vi "Check AI IRQ.vi"(5 "Hysteresis":u16, 6 "FIFO In":refnum<k21>="IRQ Queue", 7 "IRQ Number":u8, 8 "Threshold":u16, 9 "Analog Value":u16, 10 "Rising Edge?":bool, 11 "Enable Interrupt?":bool) -> ()   [LabVIEW 2017]
doc: "This VI checks if the analog input interrupt is triggered under the specified condition.\n<b>IRQ Number</b> specifies the identifier of the interrupt. <b>IRQ Number</b> ranges from 1 to 8 on FPGA and is shared between analog, digital, and button interrupts."
uses:
  <vilib>/Platform/TimedLoop/XDataNode/timing_clust.ctl
  <vilib>/Platform/TimedLoop/XDataNode/nitl_modes.ctl
  <vilib>/Platform/TimedLoop/XDataNode/wakeup.ctl
  <vilib>/rvi/Emulation/niFpgaSctlEmulationGetInTimedLoop.vi
  <vilib>/rvi/Emulation/niFpgaEmulationReportErrorSimple.vi
  <vilib>/rvi/Emulation/niFpgaGetClockAttributes.vi
  <vilib>/rvi/Emulation/niFpgaCriticalErrorInLSC.vi
  <vilib>/rvi/DataTransferAndStorage/Container/Common/niFpgaContainerExecOnDevCompGetState.vi
  <vilib>/rvi/Emulation/niFpgaEmulationIsFPGAContextNoSignature.vi
  <vilib>/rvi/errors/niFpgaSetErrorForExecOnDevCompSimple.vi
  <vilib>/rvi/eio/common/nirviEmuReportErrorAndStop.vi
  <vilib>/rvi/DataTransferAndStorage/Container/Common/niFpgaContainerGetUniqueNameForEmu.vi
  <vilib>/rvi/FIFO/Fifo_Resource/nirvififoEmulationSetSize.vi
  <vilib>/rvi/FIFO/Fifo_Resource/nirviFifoEmulationQueueMgr.vi
  <instcachedir>/0/nirviFifoEmulationQueueMgr_E5CAEC123FF24DC58D834DCA3CDAA9B5.lvgen/nirviFifoEmulationQueueMgr_E5CAEC123FF24DC58D834DCA3CDAA9B5_001.vi
  <vilib>/rvi/FIFO/Fifo_Resource/nirvififoEmulationDetermineInputValidOut.vi
  <vilib>/rvi/FIFO/Fifo_Resource/nirvififoEmulationCreateLock.vi
  <vilib>/rvi/Emulation/niFpgaProcessEmulError.vi
  <vilib>/rvi/FIFO/Fifo_Resource/nirvififoEmulationObtainLock.vi
  <vilib>/rvi/FIFO/Fifo_Resource/nirvififoEmulationReleaseLock.vi
  <vilib>/rvi/occurrence/nirviWaitOnOccurrenceBase.vi
  <vilib>/rvi/errors/nirviReportUnexpectedCaseInternalError.vi
  <vilib>/rvi/errors/nirviReportUnexpectedCaseInternalError (U32).vi
  <vilib>/Utility/error.llb/Clear Errors.vi
  <vilib>/rvi/interface/RandomDataEmulation/niFpgaRandomDataHandleErrors.vi
  <vilib>/platform/TimedLoop/XDataNode/XDataNode.xnode
  <vilib>/rvi/DataTransferAndStorage/Container/XNode/niFpgaContainer.xnode
  <vilib>/rvi/FIFO/Fifo_Resource/niFpgaFifoEmulationRefIn.vi
  <vilib>/Platform/TimedLoop/XDataNode/XDNodeRunTimeDep.lvlib
panel:
  # "This VI checks if the analog input interrupt is triggered under the specified condition.\nIRQ Number specifies the identifier of the interrupt. IRQ Number ranges from 1 to 8 on FPGA and is shared between analog, digital, and button interrupts."
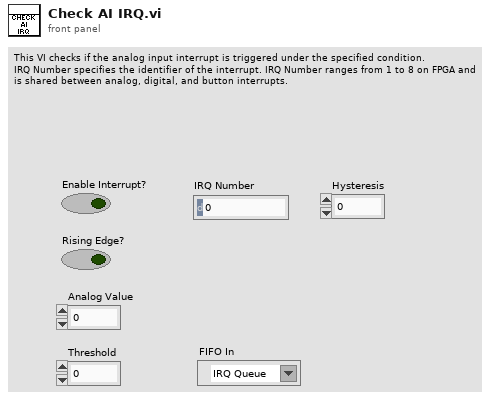
[diagram p1: front panel]
types:
  T1 = typedef "XDNodeRunTimeDep.lvlib/timing_clust.ctl" = cluster{"Expected End [f-1]":u64, "Actual End [f-1]":u64, "Finished Late? [f-1]":bool, "Expected End [i-1]":u64, "Actual End [i-1]":u64, "Finished Late? [i-1]":bool, "Expected Start [i]":u64, "Actual Start [i]":u64, "Expected Start [f]":u64, "Actual Start [f]":u64, "Source Name":string, "Structure Name":string, "Period":i64, "Deadline":i64, "Offset":i64, "Start":i64, "Priority":i32, "Timeout":i32, "Mode":T2, "Wakeup Reason":T3, "Error":errorcluster, "Source Type":string, "Secondary Source Type":string, "Global End Time":u64, "Global Start Time":u64, "Frame Duration":u64, "Iteration Duration":u64, "Assigned CPU":i32, "I/O Scan Engine Mode":u32}
  T2 = typedef "XDNodeRunTimeDep.lvlib/nitl_modes.ctl" = enum32{"No Change", "Process missed periods, maintain original phase", "Discard missed periods, maintain original phase", "Process missed periods, ignore original phase", "Discard missed periods, ignore original phase"}
  T3 = typedef "XDNodeRunTimeDep.lvlib/wakeup.ctl" = enum32{"Normal", "Aborted", "Asynchronous wakeup", "Timing source error", "Timed loop error", "Timeout"}
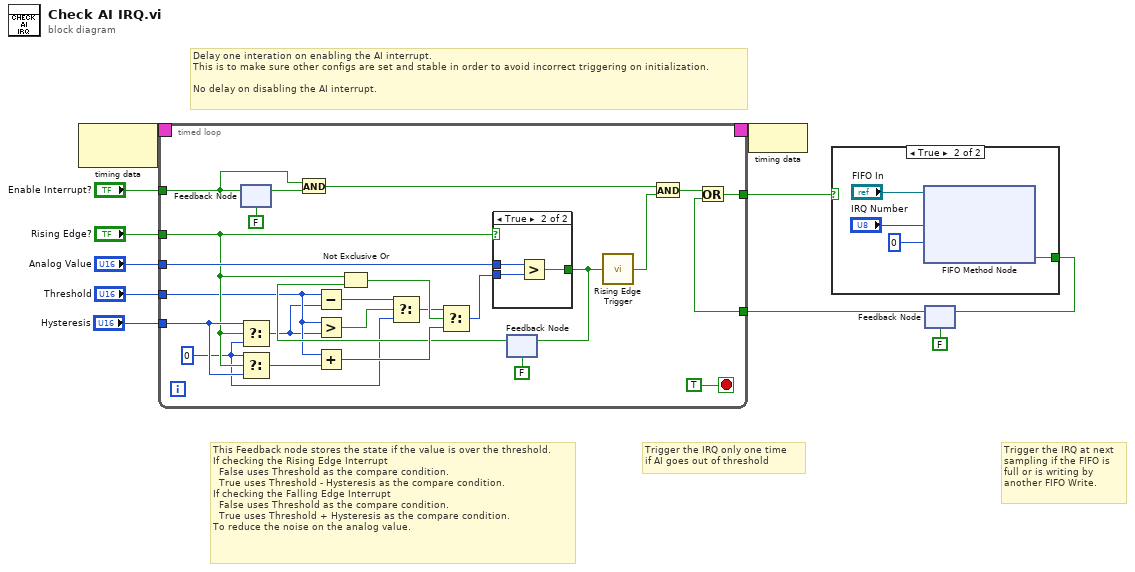
[diagram p0: block diagram]
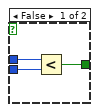
[diagram p2: hidden frame]
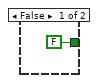
[diagram p3: hidden frame]
diagram:
  # "Delay one interation on enabling the AI interrupt.\nThis is to make sure other configs are set and stable in order to avoid incorrect triggering on initialization.\n\nNo delay on disabling the AI interrupt."
  # "Trigger the IRQ only one time \nif AI goes out of threshold"
  # "This Feedback node stores the state if the value is over the threshold.\nIf checking the Rising Edge Interrupt\n  False uses Threshold as the compare condition.\n  True uses Threshold - Hysteresis as the compare condition.\nIf checking the Falling Edge Interrupt\n  False uses Threshold as the compare condition.\n  True uses Threshold + Hysteresis as the compare condition.\nTo reduce the noise on the analog value."
  # "Trigger the IRQ at next \nsampling if the FIFO is \nfull or is writing by \nanother FIFO Write."
  n1 = node-c288() -> (w7:T1)  [unwired: 1 in]
  n2 = feedback #1(FALSE ("Timed Out?")) -> (w2:bool)
  n3 = timed-loop {
    timing: w7 -> [_]
    timing-out: [_] -> w6
    tunnel: "Analog Value" -> [w36]
    tunnel: "Threshold" -> [w23]
    tunnel: "Hysteresis" -> [w26]
    tunnel: "Rising Edge?" -> [w25]
    tunnel: [w28] -> w3
    tunnel: w2 -> [w27]
    tunnel: "Enable Interrupt?" -> [w15]
    stop <- TRUE stop-if-true
    w18 = u16 0 ("f")
    n4 = feedback-in #2(w15) -> ()
    n5 = feedback #2(FALSE ("Enable Interrupt?")) -> (w14:bool)
    n6 = Select(t=w26, s=w25, f=w18) -> (s? t:f=w22:u16)
    n7 = Select(t=w18, s=w25, f=w26) -> (s? t:f=w24:u16)
    n8 = And(x=w15, y=w14) -> (x .and. y?=w13:bool)
    n9 = Subtract(x=w23, y=w22) -> (x-y=w20:u16)
    n10 = Greater?(x=w23, y=w22) -> (0:w21:bool)
    n11 = Add(x=w23, y=w24) -> (x+y=w34:u16)
    n12 = Select(t=w20, s=w21, f=w18) -> (s? t:f=w19:u16)
    n13 = feedback #3(FALSE ("Timed Out?")) -> (w31:bool)
    n14 = Not Exclusive Or(1:w31, 2:w25) -> (0:w30:bool)
    n15 = Select(t=w19, s=w30, f=w34) -> (s? t:f=w33:u16)
    n16 = case shown="True" w25 {
      tunnel: w36 -> [w39 w42]
      tunnel: w33 -> [w38 w41]
      tunnel: [w37 w40] -> w32
      frame False {
        n17 = Less?(x=w39, y=w38) -> (x < y?=w37:bool)
      }
      frame True {
        n18 = Greater?(x=w42, y=w41) -> (0:w40:bool)
      }
    }
    n19 = feedback-in #3(w32) -> ()
    n20 = call "Rising Edge Trigger.vi"("Signal"=w32) -> ("Trigger?"=w17:bool)
    n21 = And(x=w13, y=w17) -> (x .and. y?=w16:bool)
    n22 = Or(x=w16, y=w27) -> (x .or. y?=w28:bool)
  }
  n23 = node-c288(w6) -> ()
  n24 = case shown="True" w3 {
    tunnel: [FALSE ("Timed Out?") w46] -> w5
    frame False {
    }
    frame True {
      n25 = xnode ("FIFO Method Node")("Element"="IRQ Number", "Timeout"=0, "FIFO In"="FIFO In") -> ("Timed Out?"=w46:bool)  [unwired: 1 out]
    }
  }
  n26 = feedback-in #1(w5) -> ()
